vi "N330X Acquire Voltage and Current Measurement no enable.vi"() -> ()   [LabVIEW 2015]
doc: "This example shows how to acquire a measurement.\n\n<B>Note:</B>\nTo run this example successfully, connect the Load to a DC power supply in Constant Voltage (CV) mode."
panel:
  out "Maximum Voltage":dbl
  out "Minimum Voltage":dbl
  out "Total RMS Voltage":dbl
  out "Input Voltage":dbl
  out "Input Current":dbl
  in  "Trigger Source (2: Hold)":i32(ring)=2 items=["Bus", "External", "Hold", "Line", "Timer"]
  in  "Current Measurement Range (0 A)":dbl=1.0
  in  "Triggered Current Level (0 A)":dbl=1.0
  in  "Input Current (0 A)":dbl=1.0
  in  "Input Current Range":dbl=1.0
  in  "Regulator (0:Fixed)":i32(ring) items=["Fixed", "List"]
  in  "Regulation Mode (0:Current)":i32(ring) items=["Current", "Resistance", "Voltage"]
  in  "Channel (1)":u32=1
  out "Maximum Current":dbl
  out "Minimum Current":dbl
  out "Total RMS Current":dbl
  in  "VISA resource name":refnum<visa-resource-name>
  # "(c) 2007-2015 National Instruments.  ALL RIGHTS RESERVED."
  # "To run this Example, connect\nthe Load to a DC power supply\nin Constant Voltage Mode"
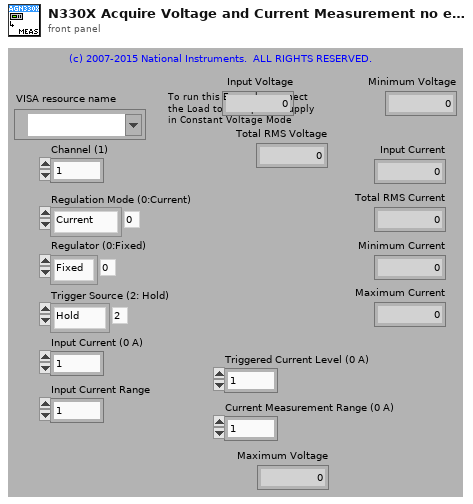
[diagram p1: front panel]
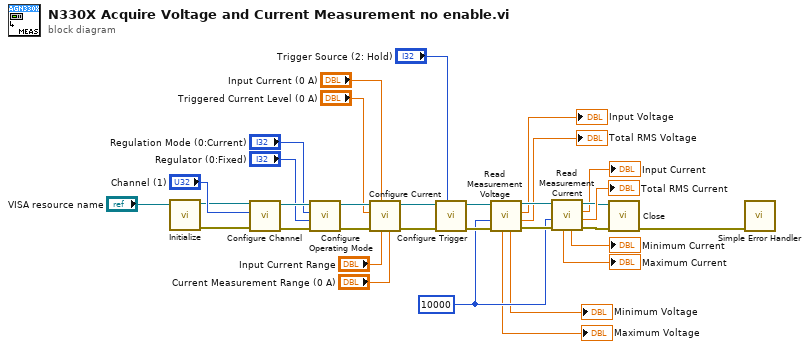
[diagram p0: block diagram]
diagram:
  w5 = u32 10000 ("Maximum Time (5000 ms)")
  n1 = call <instrlib>:"Initialize.vi"("VISA resource name"="VISA resource name") -> ("error out"=w19:errorcluster, "VISA resource name out"=w20:refnum<visa-resource-name>)  [unwired: 9 in]
  n2 = call <instrlib>:"Configure Channel.vi"("error in (no error)"=w19, "Channel (1)"="Channel (1)", "VISA resource name"=w20) -> ("error out"=w31:errorcluster, "VISA resource name out"=w33:refnum<visa-resource-name>)  [unwired: 7 in]
  n3 = call <instrlib>:"Configure Operating Mode.vi"("error in (no error)"=w31, "Regulator (0:Fixed)"="Regulator (0:Fixed)", "Regulation Mode (0:Current)"="Regulation Mode (0:Current)", "VISA resource name"=w33) -> ("error out"=w30:errorcluster, "VISA resource name out"=w32:refnum<visa-resource-name>)  [unwired: 6 in]
  n4 = call <instrlib>:"Configure Current.vi"("Current Measurement Range (1 A)"="Current Measurement Range (0 A)", "Input Current Range (1 A)"="Input Current Range", "Input Current (1 A)"="Input Current (0 A)", "error in (no error)"=w30, "Triggered Current Level (1 A)"="Triggered Current Level (0 A)", "VISA resource name"=w32) -> ("error out"=w22:errorcluster, "VISA resource name out"=w23:refnum<visa-resource-name>)  [unwired: 4 in]
  n5 = call <instrlib>:"Configure Trigger.vi"("Trigger Source (2: Hold)"="Trigger Source (2: Hold)", "error in (no error)"=w22, "VISA resource name"=w23) -> ("error out"=w8:errorcluster, "VISA resource name out"=w9:refnum<visa-resource-name>)  [unwired: 7 in]
  n6 = call <instrlib>:"Read Measurement Voltage.vi"("error in (no error)"=w8, "Maximum Time (10000 ms)"=w5, "VISA resource name"=w9) -> ("error out"=w6:errorcluster, "Total RMS Voltage"=→"Total RMS Voltage":dbl, "Input Voltage"=→"Input Voltage":dbl, "VISA resource name out"=w7:refnum<visa-resource-name>, "Minimum Voltage"=→"Minimum Voltage":dbl, "Maximum Voltage"=→"Maximum Voltage":dbl)  [unwired: 3 in]
  n7 = call <instrlib>:"Read Measurement Current.vi"("error in (no error)"=w6, "Maximum Time (10000 ms)"=w5, "VISA resource name"=w7) -> ("error out"=w17:errorcluster, "Total RMS Current"=→"Total RMS Current":dbl, "Input Current"=→"Input Current":dbl, "VISA resource name out"=w18:refnum<visa-resource-name>, "Minimum Current"=→"Minimum Current":dbl, "Maximum Current"=→"Maximum Current":dbl)  [unwired: 3 in]
  n8 = call <instrlib>:"Close.vi"("error in (no error)"=w17, "VISA resource name"=w18) -> ("error out"=w16:errorcluster)  [unwired: 9 in]
  n9 = call <vilib>:"Simple Error Handler.vi"("error in (no error)"=w16) -> ()  [unwired: 4 in, 5 out]
